vi "LEP_RV_UVAddOptions.vi"(0 "Config":T1 {"Constant Deallocation" items=["Out of Scope", "VI End", "Application End"]; "Constant Allocation" items=["First Use", "Containing Loop", "VI Initialization", "Application Initialization"]; "Target serial port" items=["0", "1", "2", "3"]; "Console output" items=["Processor status window", "Serial port"]; "Optimization" items=["Level 0 (-O0)", "Level 1 (-O1)", "Level 2 (-O2)", "Level 3 (-O3)"]; "Mode" items=["ARM-Mode", "Thumb-Mode"]; "Debug Options" items=["Use ULINK Debugger", "Use Simulator"]; "Debug Mode" items=["Instrumented (serial port)", "Instrumented (TCP/IP)", "Non-instrumented (JTAG/USB)"]}, 1 "Target":string, 2 "VI Group Name":string="VIs", 3 "LV Runtime Group Name":string="Runtime", 4 "Path to VI Files":path=path "../../../..", 5 "error in (no error)":errorcluster, 7 "Drivers Group Name":string="VIs", 9 "uVision Project":path) -> (19 "error out":errorcluster)   [LabVIEW 2011]
doc: "Runs the embedded application on a console located in the <B>Build Path</B> directory ."
uses:
  LEP_RV_Config.ctl
  <vilib>/Platform/EmbProject/Plugins/utilities/LEP_Utilities_GetSetProjectData_Variant.vi
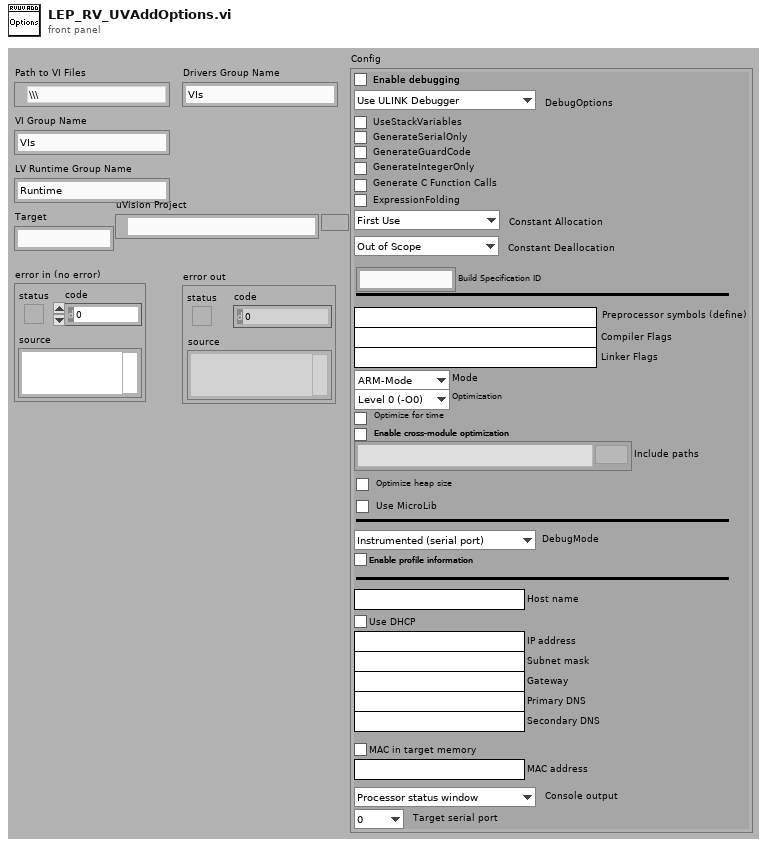
[diagram p1: front panel]
types:
  T1 = typedef "LEP_RV_Config.ctl" = cluster{"Enable debugging":bool, "Debug Options":u16, "Use stack variables":bool, "Generate serial only":bool, "Generate guard code":bool, "Generate Integer Only":bool, "Generate C Function Calls":bool, "ExpressionFolding":bool, "Constant Allocation":u16, "Constant Deallocation":u16, "Build Specification ID":string, "Preprocessor symbols (define)":string, "Compiler Flags":string, "Linker Flags":string, "Mode":u16, "Optimization":u16, "Optimize for time":bool, "Enable cross-module optimization":bool, "Include paths":path[], "Optimize heap size":bool, "Use MicroLib":bool, "Debug Mode":u16, "Enable profile information":bool, "Host name":string, "Use DHCP":bool, "IP address":string, "Subnet mask":string, "Gateway":string, "Primary DNS":string, "Secondary DNS":string, "MAC in target memory":bool, "MAC address":string, "Console output":u16, "Target serial port":u16}
  T2 = enum32{"Unused", "OPT_LMISC", "OPT_CMISC", "OPT_AMISC", "OPT_CINCL", "OPT_AINCL", "OPT_CDEF", "OPT_ADEF", "OPT_CUNDEF", "OPT_AUNDEF"}
  T3 = enum32{"Unused", "OPT_LMISC", "OPT_CMISC", "OPT_AMISC", "OPT_CINCL", "OPT_AINCL", "OPT_CDEF", "OPT_ADEF", "OPT_CUNDEF", "OPT_AUNDEF", "OPT_COPTIMIZE", "OPT_CODEGEN", "OPT_MEMRANGES"}
  T4 = enum32{"Unused", "OPT_LMISC", "OPT_CMISC", "OPT_AMISC", "OPT_CINCL", "OPT_AINCL", "OPT_CDEF", "OPT_ADEF", "OPT_CUNDEF", "OPT_AUNDEF", "OPT_COPTIMIZE", "OPT_CODEGEN", "OPT_MEMRANGES", "OPT_ASNMEMRANGES"}
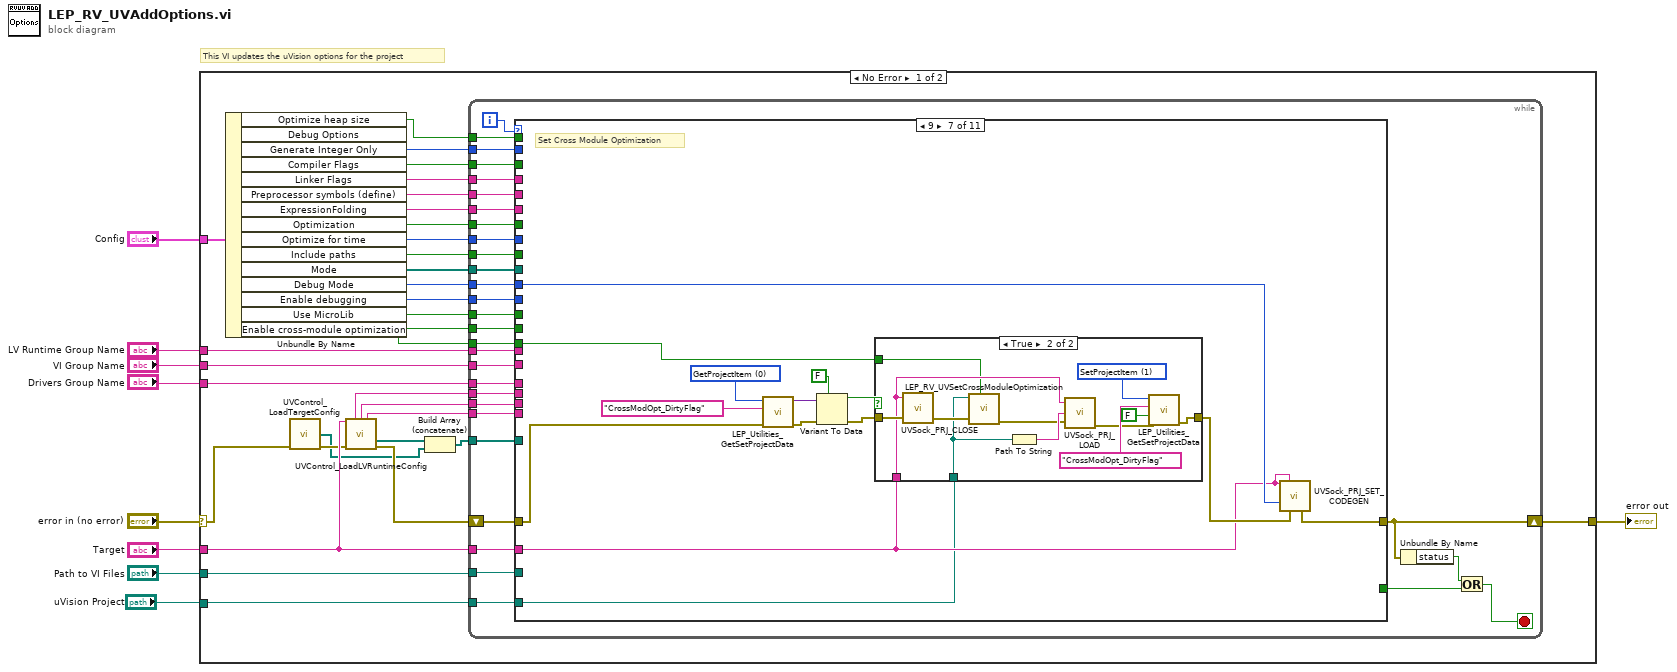
[diagram p0: block diagram]
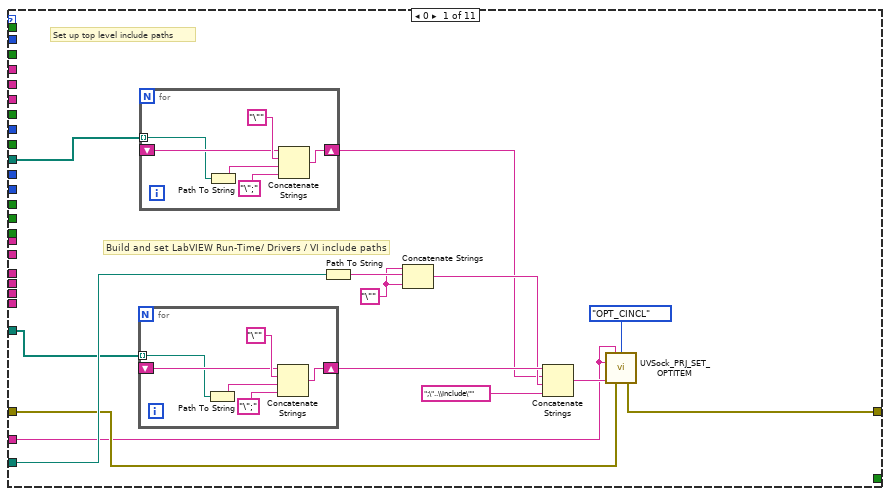
[diagram p2: hidden frame]
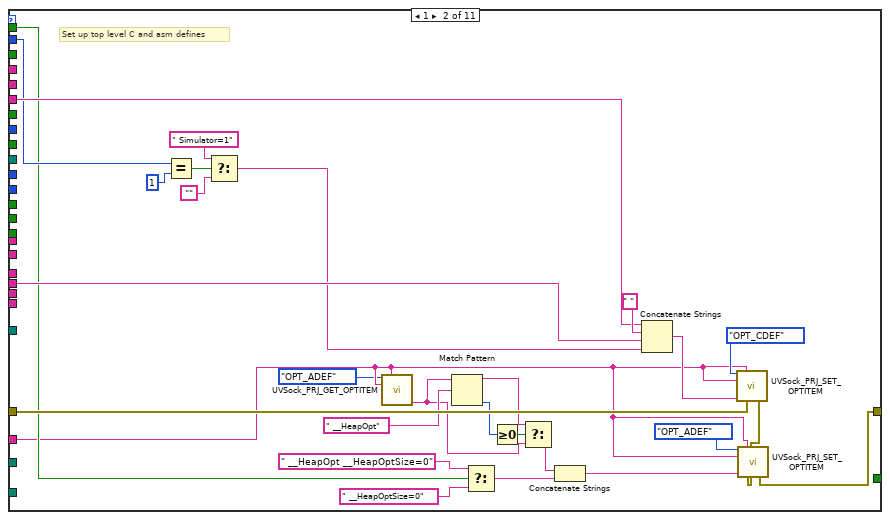
[diagram p3: hidden frame]
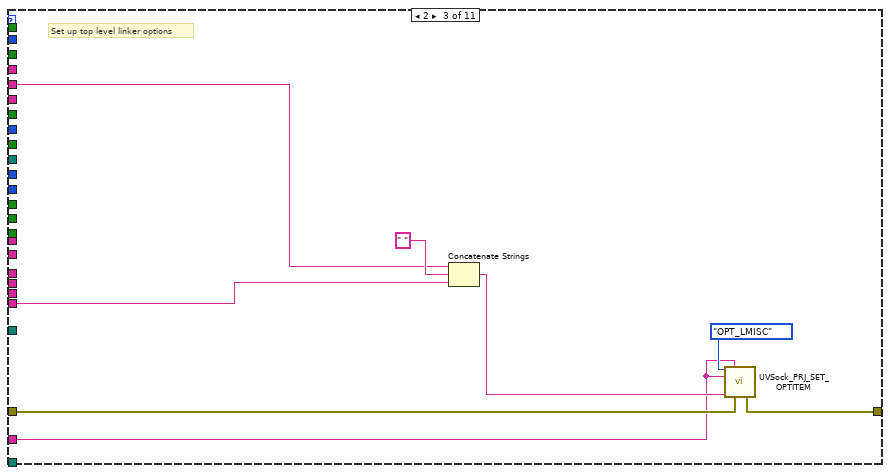
[diagram p4: hidden frame]
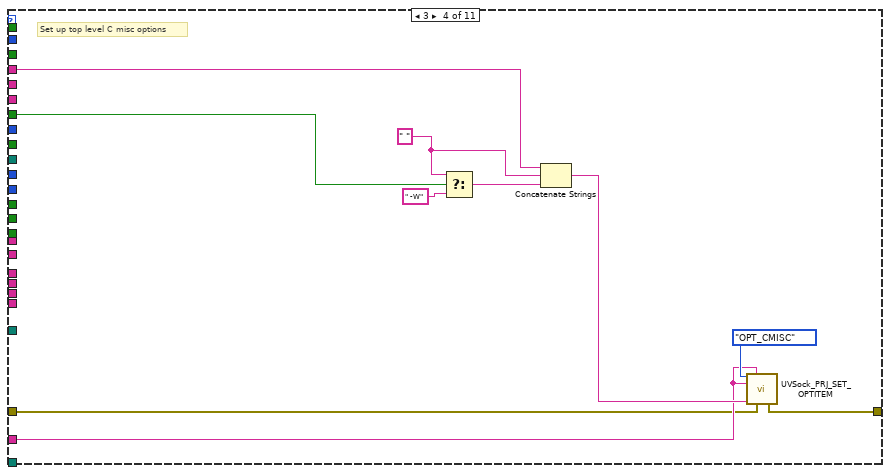
[diagram p5: hidden frame]
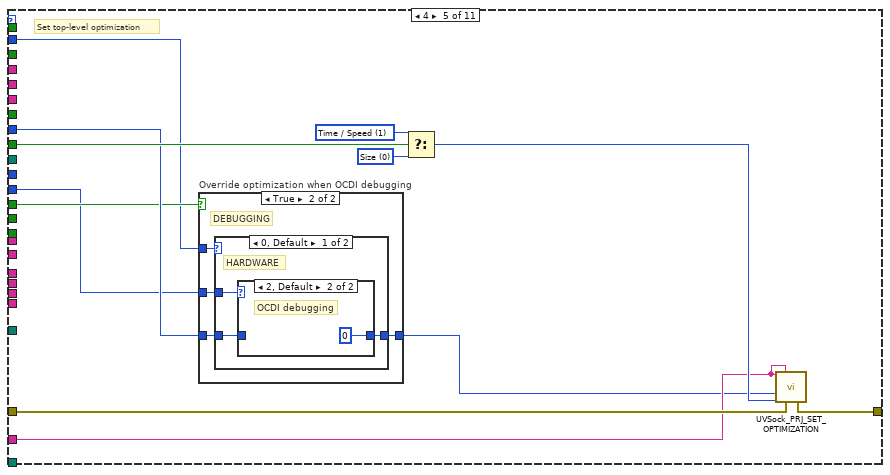
[diagram p6: hidden frame]
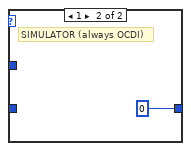
[diagram p9: hidden frame]
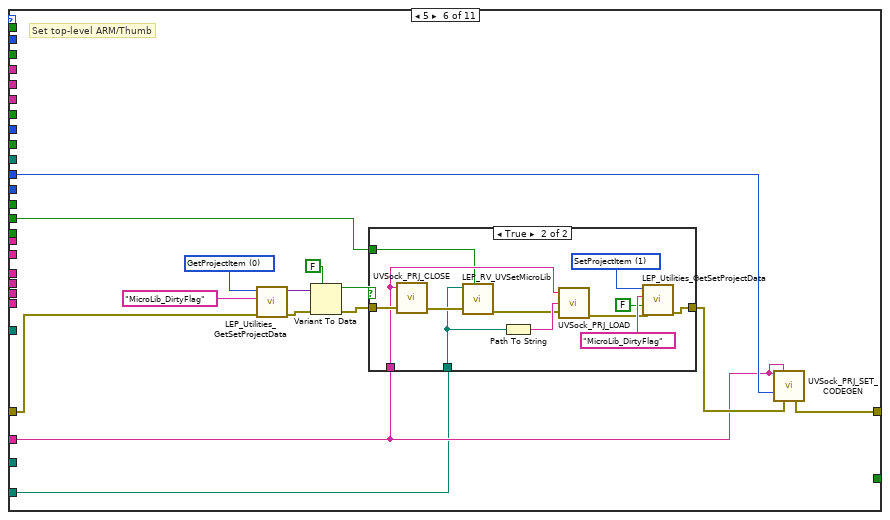
[diagram p10: hidden frame]
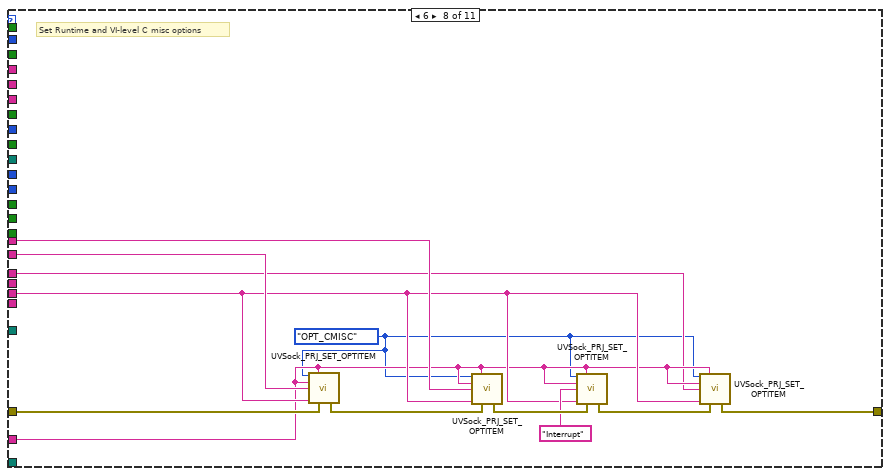
[diagram p13: hidden frame]
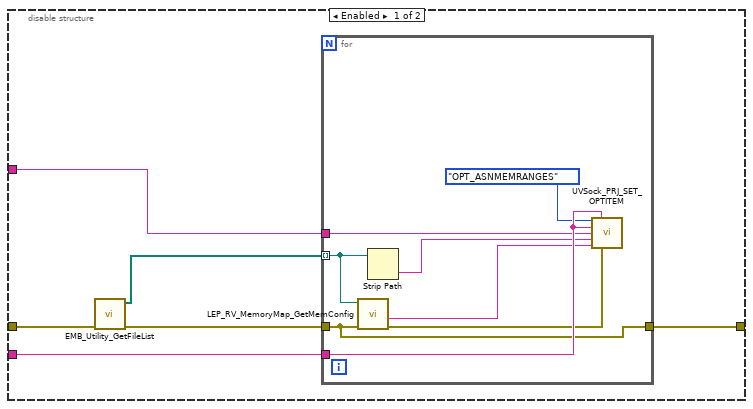
[diagram p15: hidden frame]
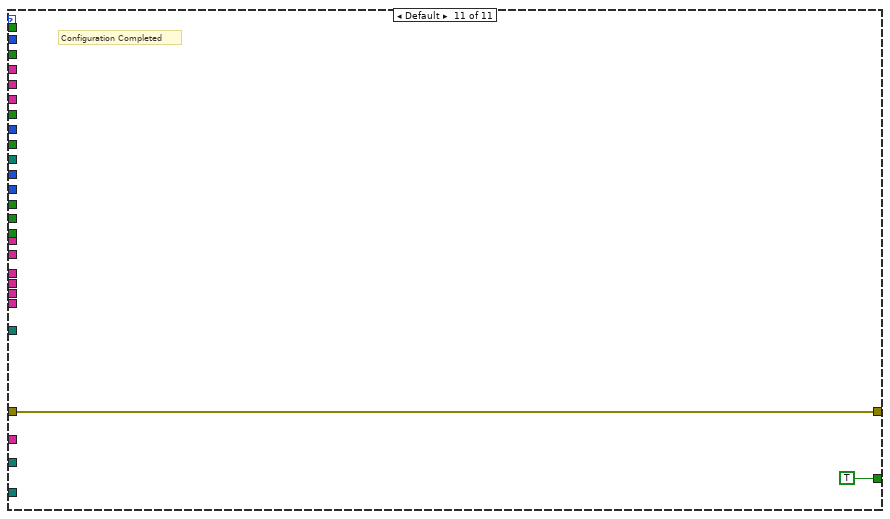
[diagram p17: hidden frame]
diagram:
  # "This VI updates the uVision options for the project"
  n1 = case shown="No Error" "error in (no error)" {
    selector: "error in (no error)" -> [w15 w254]
    tunnel: "Config" -> [w22 _]
    tunnel: [w28 w254] -> w5
    tunnel: "Target" -> [w27 _]
    tunnel: "Path to VI Files" -> [w26 _]
    tunnel: "LV Runtime Group Name" -> [w24 _]
    tunnel: "VI Group Name" -> [w23 _]
    tunnel: "Drivers Group Name" -> [w16 _]
    tunnel: "uVision Project" -> [w11 _]
    frame No Error {
      n2 = Unbundle By Name(w22) -> ("Optimize heap size"=w13:bool, "Debug Options"=w21:u16, "Generate Integer Only"=w25:bool, "Compiler Flags"=w39:string, "Linker Flags"=w38:string, "Preprocessor symbols (define)"=w37:string, "ExpressionFolding"=w36:bool, "Optimization"=w35:u16, "Optimize for time"=w34:bool, "Include paths"=w40:path[], "Mode"=w33:u16, "Debug Mode"=w32:u16, "Enable debugging"=w14:bool, "Use MicroLib"=w12:bool, "Enable cross-module optimization"=w10:bool)
      n3 = call "UVControl_LoadTargetConfig.vi"("error in (no error)"=w15) -> ("Driver Include Paths"=w17:path[], "error out"=w20:errorcluster)  [unwired: 9 in, 4 out]
      n4 = call "UVControl_LoadLVRuntimeConfig.vi"("Target"=w27, "error in (no error)"=w20) -> ("Defines"=w29:string, "Compiler Misc Controls"=w30:string, "Linker Misc Controls"=w31:string, "RunTime Include Paths"=w18:path[], "error out"=w41:errorcluster)  [unwired: 8 in, 1 out]
      n5 = Build Array (concatenate)(w18, w17) -> (w19:path[])
      n6 = while {
        tunnel: w19 -> [w72]
        tunnel: w27 -> [w71]
        tunnel: w26 -> [w70]
        shift-right: [w65] -> w28
        shift-left: w41 -> [w64]
        tunnel: w40 -> [w63]
        tunnel: w39 -> [w62]
        tunnel: w38 -> [w61]
        tunnel: w37 -> [w60]
        tunnel: w36 -> [w59]
        tunnel: w35 -> [w58]
        tunnel: w34 -> [w57]
        tunnel: w33 -> [w56]
        tunnel: w32 -> [w55]
        tunnel: w31 -> [w54]
        tunnel: w30 -> [w53]
        tunnel: w29 -> [w52]
        tunnel: w25 -> [w51]
        tunnel: w24 -> [w50]
        tunnel: w23 -> [w49]
        tunnel: w21 -> [w48]
        tunnel: w16 -> [w47]
        tunnel: w14 -> [w46]
        tunnel: w13 -> [w45]
        tunnel: w12 -> [w44]
        tunnel: w11 -> [w43]
        tunnel: w10 -> [w42]
        i -> [w69]
        stop <- w66 stop-if-true
        n7 = case shown="9" w69 {
          tunnel: w71 -> [w73 w108 w127 w137 w150 w169 w196 w222 w234 _ _]
          tunnel: w70 -> [w80 _ _ _ _ _ _ _ _ _ _]
          tunnel: w72 -> [w79 _ _ _ _ _ _ _ _ _ _]
          tunnel: [_ _ _ _ _ _ _ _ _ _ TRUE] -> w67
          tunnel: [w76 w113 w133 w143 w156 w181 w207 w224 w235 w251 w252] -> w65
          tunnel: w64 -> [w75 w124 w132 w135 w155 w177 w203 w229 w233 w251 w252]
          tunnel: w63 -> [w74 _ _ _ _ _ _ _ _ _ _]
          tunnel: w62 -> [_ _ _ w139 _ _ _ _ _ _ _]
          tunnel: w61 -> [_ _ w130 _ _ _ _ _ _ _ _]
          tunnel: w60 -> [_ w122 _ _ _ _ _ _ _ _ _]
          tunnel: w59 -> [_ _ _ w141 _ _ _ _ _ _ _]
          tunnel: w58 -> [_ _ _ _ w149 _ _ _ _ _ _]
          tunnel: w57 -> [_ _ _ _ w152 _ _ _ _ _ _]
          tunnel: w56 -> [_ _ _ _ _ w180 w206 _ _ _ _]
          tunnel: w55 -> [_ _ _ _ w145 _ _ _ _ _ _]
          tunnel: w54 -> [_ _ w129 _ _ _ _ _ _ _ _]
          tunnel: w53 -> [_ _ _ _ _ _ _ w223 _ _ _]
          tunnel: w52 -> [_ w121 _ _ _ _ _ _ _ _ _]
          tunnel: w51 -> [_ _ _ _ _ _ _ _ _ _ _]
          tunnel: w50 -> [_ _ _ _ _ _ _ w230 _ _ _]
          tunnel: w49 -> [_ _ _ _ _ _ _ w231 w232 _ _]
          tunnel: w48 -> [_ w116 _ _ w146 _ _ _ _ _ _]
          tunnel: w47 -> [_ _ _ _ _ _ _ w221 _ _ _]
          tunnel: w46 -> [_ _ _ _ w147 _ _ _ _ _ _]
          tunnel: w45 -> [_ w112 _ _ _ _ _ _ _ _ _]
          tunnel: w44 -> [_ _ _ _ _ w170 _ _ _ _ _]
          tunnel: w43 -> [_ _ _ _ _ w168 w195 _ _ _ _]
          tunnel: w42 -> [_ _ _ _ _ _ w194 _ _ _ _]
          frame 0 {
            w82 = "\"" ("string")
            # "Build and set LabVIEW Run-Time/ Drivers / VI include paths"
            # "Set up top level include paths"
            n8 = for {
              tunnel: w79 -> [w93] mode=indexing
              shift-right: [w98] -> w86
              shift-left: _ -> [w94]
              n9 = Path To String(path=w93) -> (string=w97:string)
              n10 = Concatenate Strings(w94, "\"" ("string"), w97, "\";" ("string")) -> (w98:string)
            }
            n11 = for {
              tunnel: w74 -> [w87] mode=indexing
              shift-right: [w92] -> w78
              shift-left: _ -> [w88]
              n12 = Path To String(path=w87) -> (string=w91:string)
              n13 = Concatenate Strings(w88, "\"" ("string"), w91, "\";" ("string")) -> (w92:string)
            }
            n14 = Path To String(path=w80) -> (string=w83:string)
            n15 = Concatenate Strings(w82, w83, w82) -> (w81:string)
            n16 = Concatenate Strings(w86, w78, w81, ";\"..\\Include\"" ("string")) -> (w85:string)
            n17 = call "UVSock_PRJ_SET_OPTITEM.vi"("Option In"=T2."OPT_CINCL", "Target"=w73, "Target Name In"=w73, "Item In"=w85, "error in (no error)"=w75) -> ("error out"=w76:errorcluster)  [unwired: 10 in]
          }
          frame 1 {
            # "Set up top level C and asm defines"
            n18 = Equal?(x=w116, y=u16 1) -> (x = y?=w118:bool)
            n19 = Select(t=" Simulator=1", s=w118, f="") -> (s? t:f=w115:string)
            n20 = call "UVSock_PRJ_GET_OPTITEM.vi"("Option In"=T3."OPT_ADEF", "Target"=w108, "Target Name In"=w108) -> ("Item Out"=w101:string)  [unwired: 10 in, 2 out]
            n21 = Match Pattern(string=w101, regular expression=" __HeapOpt") -> (before substring=w100:string, offset past match=w102:i32)  [unwired: 1 in, 2 out]
            n22 = Select(t=" __HeapOpt __HeapOptSize=0" ("string"), s=w112, f=" __HeapOptSize=0") -> (s? t:f=w105:string)
            n23 = Greater Or Equal To 0?(x=w102) -> (x >= 0?=w103:bool)
            n24 = Select(t=w100, s=w103, f=w101) -> (s? t:f=w99:string)
            n25 = Concatenate Strings(w99, w105) -> (w106:string)
            n26 = Concatenate Strings(w122, " " ("string"), w121, w115) -> (w125:string)
            n27 = call "UVSock_PRJ_SET_OPTITEM.vi"("Option In"=T2."OPT_CDEF", "Target"=w108, "Target Name In"=w108, "Item In"=w125, "error in (no error)"=w124) -> ("error out"=w114:errorcluster)  [unwired: 10 in]
            n28 = call "UVSock_PRJ_SET_OPTITEM.vi"("Option In"=T4."OPT_ADEF", "Target"=w108, "Target Name In"=w108, "Item In"=w106, "error in (no error)"=w114) -> ("error out"=w113:errorcluster)  [unwired: 10 in]
          }
          frame 2 {
            # "Set up top level linker options"
            n29 = Concatenate Strings(w130, " " ("string"), w129) -> (w128:string)
            n30 = call "UVSock_PRJ_SET_OPTITEM.vi"("Option In"=T2."OPT_LMISC", "Target"=w127, "Target Name In"=w127, "Item In"=w128, "error in (no error)"=w132) -> ("error out"=w133:errorcluster)  [unwired: 10 in]
          }
          frame 3 {
            w136 = " " ("string")
            # "Set up top level C misc options"
            n31 = Select(t=w136, s=w141, f=" -W") -> (s? t:f=w138:string)
            n32 = Concatenate Strings(w139, w136, w138) -> (w140:string)
            n33 = call "UVSock_PRJ_SET_OPTITEM.vi"("Option In"=T2."OPT_CMISC", "Target"=w137, "Target Name In"=w137, "Item In"=w140, "error in (no error)"=w135) -> ("error out"=w143:errorcluster)  [unwired: 10 in]
          }
          frame 4 {
            w153 = 1 items=["<default>"=-1, "Size"=0, "Time / Speed"=1] ("Optimize Type")
            w154 = 0 items=["<default>"=-1, "Size"=0, "Time / Speed"=1] ("Optimize Type")
            # "Set top-level optimization"
            n34 = case "Override optimization when OCDI debugging" shown="True" w147 {
              tunnel: w149 -> [w157 w161]
              tunnel: [w157 w160] -> w148
              tunnel: w146 -> [_ w159]
              tunnel: w145 -> [_ w158]
              frame False {
                # "NOT DEBUGGING"
              }
              frame True {
                # "DEBUGGING"
                n35 = case shown="0, Default" w159 {
                  tunnel: w161 -> [w164 _]
                  tunnel: [w163 u16 0 ("Optimization")] -> w160
                  tunnel: w158 -> [w162 _]
                  frame 0, Default {
                    # "HARDWARE"
                    n36 = case shown="2, Default" w162 {
                      tunnel: w164 -> [w165 _]
                      tunnel: [w165 u16 0 ("Optimization")] -> w163
                      frame 0, 1 {
                        # "INSTR debugging"
                      }
                      frame 2, Default {
                        # "OCDI debugging"
                      }
                    }
                  }
                  frame 1 {
                    # "SIMULATOR (always OCDI)"
                  }
                }
              }
            }
            n37 = Select(t=w153, s=w152, f=w154) -> (s? t:f=w151:i32)
            n38 = call "UVSock_PRJ_SET_OPTIMIZATION.vi"("Target Name"=w150, "Target"=w150, "Optimization Level"=w148, "Optimize Type"=w151, "error in (no error)"=w155) -> ("error out"=w156:errorcluster)  [unwired: 10 in]
          }
          frame 5 {
            w178 = u16 0 items=["GetProjectItem", "SetProjectItem"] ("Command")
            # "Set top-level ARM/Thumb"
            n39 = call-poly <vilib>:"LEP_Utilities_GetSetProjectData.vi"("error in"=w177, "ItemName"="MicroLib_DirtyFlag", "Command"=w178) -> ("error out"=w176:errorcluster, "Variant Out"=w175:variant)  [unwired: 3 in, 4 out]
            n40 = Variant To Data(error in=w176, type=FALSE, Variant=w175) -> (data=w173:bool, error out=w172:errorcluster)
            n41 = case shown="True" w173 {
              tunnel: w172 -> [_ w188]
              tunnel: [_ w191] -> w171
              tunnel: w170 -> [_ w182]
              tunnel: w169 -> [_ w186]
              tunnel: w168 -> [_ w183]
              frame False {
              }
              frame True {
                w193 = u16 1 items=["GetProjectItem", "SetProjectItem"] ("Command")
                n42 = call "UVSock_PRJ_CLOSE.vi"("error in (no error)"=w188, "Target"=w186) -> ("error out"=w185:errorcluster)  [unwired: 3 in]
                n43 = call "LEP_RV_UVSetMicroLib.vi"("Use MicroLib"=w182, "error in (no error)"=w185, "uVision Project"=w183) -> ("error out"=w184:errorcluster)  [unwired: 8 in]
                n44 = Path To String(path=w183) -> (string=w187:string)
                n45 = call "UVSock_PRJ_LOAD.vi"("error in (no error)"=w184, "Project File"=w187, "Target"=w186) -> ("error out"=w189:errorcluster)  [unwired: 2 in]
                n46 = call-poly <vilib>:"LEP_Utilities_GetSetProjectData.vi"("error in"=w189, "Variant In"=FALSE, "ItemName"="MicroLib_DirtyFlag", "Command"=w193) -> ("error out"=w191:errorcluster)  [unwired: 2 in, 5 out]
              }
            }
            n47 = call "UVSock_PRJ_SET_CODEGEN.vi"("Target Name"=w169, "Target"=w169, "Code Type"=w180, "error in (no error)"=w171) -> ("error out"=w181:errorcluster)  [unwired: 11 in]
          }
          frame 9 {
            w204 = u16 0 items=["GetProjectItem", "SetProjectItem"] ("Command")
            # "Set Cross Module Optimization"
            n48 = call-poly <vilib>:"LEP_Utilities_GetSetProjectData.vi"("error in"=w203, "ItemName"="CrossModOpt_DirtyFlag", "Command"=w204) -> ("error out"=w202:errorcluster, "Variant Out"=w201:variant)  [unwired: 3 in, 4 out]
            n49 = Variant To Data(error in=w202, type=FALSE, Variant=w201) -> (data=w199:bool, error out=w198:errorcluster)
            n50 = case shown="True" w199 {
              tunnel: w198 -> [_ w214]
              tunnel: [_ w217] -> w197
              tunnel: w194 -> [_ w208]
              tunnel: w196 -> [_ w212]
              tunnel: w195 -> [_ w209]
              frame False {
              }
              frame True {
                w219 = u16 1 items=["GetProjectItem", "SetProjectItem"] ("Command")
                n51 = call "UVSock_PRJ_CLOSE.vi"("error in (no error)"=w214, "Target"=w212) -> ("error out"=w211:errorcluster)  [unwired: 3 in]
                n52 = call "LEP_RV_UVSetCrossModuleOptimization.vi"("Use Cross Module Optimization"=w208, "error in (no error)"=w211, "uVision Project"=w209) -> ("error out"=w210:errorcluster)  [unwired: 8 in]
                n53 = Path To String(path=w209) -> (string=w213:string)
                n54 = call "UVSock_PRJ_LOAD.vi"("error in (no error)"=w210, "Project File"=w213, "Target"=w212) -> ("error out"=w215:errorcluster)  [unwired: 2 in]
                n55 = call-poly <vilib>:"LEP_Utilities_GetSetProjectData.vi"("error in"=w215, "Variant In"=FALSE, "ItemName"="CrossModOpt_DirtyFlag", "Command"=w219) -> ("error out"=w217:errorcluster)  [unwired: 2 in, 5 out]
              }
            }
            n56 = call "UVSock_PRJ_SET_CODEGEN.vi"("Target Name"=w196, "Target"=w196, "Code Type"=w206, "error in (no error)"=w197) -> ("error out"=w207:errorcluster)  [unwired: 11 in]
          }
          frame 6 {
            w220 = T2."OPT_CMISC" ("Option In")
            # "Set Runtime and VI-level C misc options"
            n57 = call "UVSock_PRJ_SET_OPTITEM.vi"("Option In"=w220, "Target"=w222, "Target Name In"=w222, "Group Name In"=w231, "Item In"=w223, "error in (no error)"=w229) -> ("error out"=w228:errorcluster)  [unwired: 9 in]
            n58 = call "UVSock_PRJ_SET_OPTITEM.vi"("Option In"=w220, "Target"=w222, "Target Name In"=w222, "Group Name In"=w230, "Item In"=w223, "error in (no error)"=w228) -> ("error out"=w227:errorcluster)  [unwired: 9 in]
            n59 = call "UVSock_PRJ_SET_OPTITEM.vi"("Option In"=w220, "Target"=w222, "Target Name In"=w222, "Group Name In"="Interrupt", "Item In"=w223, "error in (no error)"=w227) -> ("error out"=w225:errorcluster)  [unwired: 9 in]
            n60 = call "UVSock_PRJ_SET_OPTITEM.vi"("Option In"=w220, "Target"=w222, "Target Name In"=w222, "Group Name In"=w221, "Item In"=w223, "error in (no error)"=w225) -> ("error out"=w224:errorcluster)  [unwired: 9 in]
          }
          frame 7 {
            # "Set VI memory map options"
            n61 = disable-structure shown="Disabled" {
              disable-tunnel: [w241 w250] -> w235
              disable-tunnel: w234 -> [w240 _]
              disable-tunnel: w233 -> [w239 w250]
              disable-tunnel: w232 -> [w238 _]
              frame Enabled {
                n62 = call <vilib>:"EMB_Utility_GetFileList.vi"("error in (no error)"=w239) -> ("error out"=w237:errorcluster, "File List"=w236:path[])  [unwired: 9 in]
                n63 = for {
                  tunnel: w240 -> [w249]
                  tunnel: w238 -> [w248]
                  tunnel: w236 -> [w244] mode=indexing
                  tunnel: w237 -> [w242]
                  tunnel: [w242] -> w241
                  n64 = call "LEP_RV_MemoryMap_GetMemConfig.vi"("error in (no error)"=w242, "Source File"=w244) -> ("error out"=w246:errorcluster, "Mem Config String"=w245:string)  [unwired: 6 in, 2 out]
                  n65 = Strip Path(path=w244) -> (name=w243:string)  [unwired: 1 out]
                  n66 = call "UVSock_PRJ_SET_OPTITEM.vi"("Option In"=T4."OPT_ASNMEMRANGES", "Target"=w249, "Target Name In"=w249, "Group Name In"=w248, "File Name In"=w243, "Item In"=w245, "error in (no error)"=w246) -> ()  [unwired: 8 in, 1 out]
                }
              }
              frame Disabled {
              }
            }
          }
          frame 8 {
            # "Set Runtime and VI-level memory map options (not yet possible in LV)"
          }
          frame Default {
            # "Configuration Completed"
          }
        }
        n67 = Unbundle By Name(w65) -> ("status"=w68:bool)
        n68 = Or(x=w68, y=w67) -> (x .or. y?=w66:bool)
      }
    }
    frame Error {
    }
  }
  "error out" <- w5
